vi "Auto controll (SubVI).vi"(4 "Boolean":bool, 5 "Control Cluster in":T1 {"Yaw Speed" scale=-1.0..1.0; "Vertical Speed" scale=-1.0..1.0; "Pitch" scale=-1.0..1.0; "Roll" scale=-1.0..1.0}, 6 "Numeric":dbl, 7 "Boolean 3":bool, 8 "Boolean 4":bool, 9 "Boolean 2":bool, 10 "Number of Matches Returned":i32, 11 "Numeric 2":dbl) -> (3 "Control Cluster out":T1 {"Yaw Speed" scale=-1.0..1.0; "Vertical Speed" scale=-1.0..1.0; "Pitch" scale=-1.0..1.0; "Roll" scale=-1.0..1.0})   [LabVIEW 2014]
uses:
  Others/Control cluster.ctl
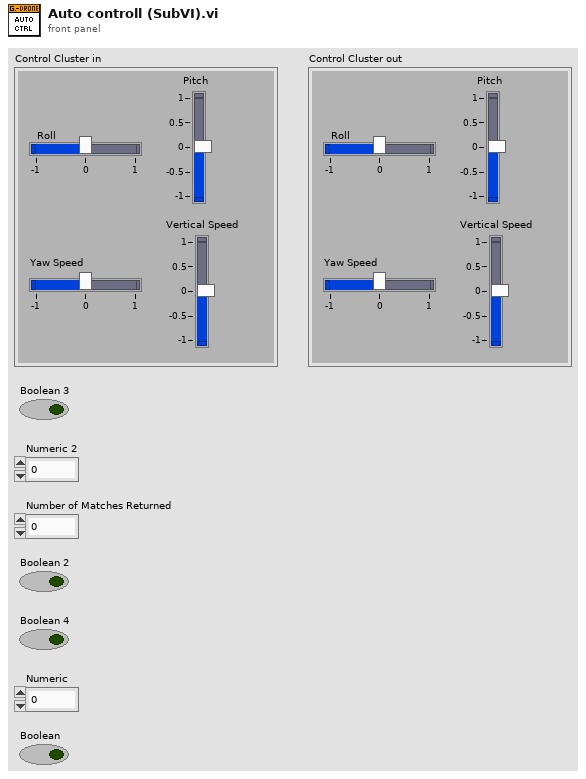
[diagram p1: front panel]
types:
  T1 = typedef "Control cluster.ctl" = cluster{"Roll":sgl, "Pitch":sgl, "Vertical Speed":sgl, "Yaw Speed":sgl}
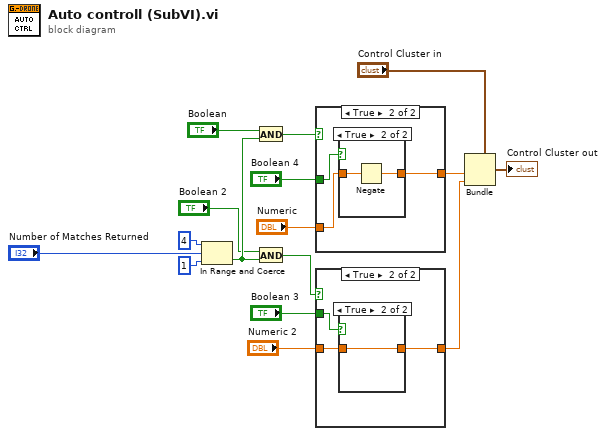
[diagram p0: block diagram]
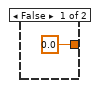
[diagram p2: hidden frame]
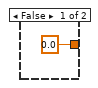
[diagram p4: hidden frame]
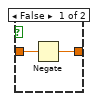
[diagram p5: hidden frame]
diagram:
  n1 = In Range and Coerce(upper limit=4, x="Number of Matches Returned", lower limit=1) -> (In Range?=w14:bool)  [unwired: 1 out]
  n2 = And(x="Boolean", y=w14) -> (x .and. y?=w13:bool)
  n3 = And(x="Boolean 2", y=w14) -> (x .and. y?=w6:bool)
  n4 = case shown="True" w13 {
    tunnel: "Boolean 4" -> [_ w20]
    tunnel: "Numeric" -> [_ w19]
    tunnel: [0.0 w18] -> w12
    frame False {
    }
    frame True {
      n5 = case shown="True" w20 {
        tunnel: w19 -> [w21 w23]
        tunnel: [w21 w22] -> w18
        frame False {
        }
        frame True {
          n6 = Negate(x=w23) -> (-x=w22:dbl)
        }
      }
    }
  }
  n7 = case shown="True" w6 {
    tunnel: "Boolean 3" -> [_ w27]
    tunnel: [0.0 w26] -> w4
    tunnel: "Numeric 2" -> [_ w25]
    frame False {
    }
    frame True {
      n8 = case shown="True" w27 {
        tunnel: w25 -> [w29 w30]
        tunnel: [w28 w30] -> w26
        frame False {
          n9 = Negate(x=w29) -> (-x=w28:dbl)
        }
        frame True {
        }
      }
    }
  }
  n10 = Bundle(cluster="Control Cluster in", "Vertical Speed"=w12, "Yaw Speed"=w4) -> (→"Control Cluster out":T1)  [unwired: 2 in]
